vi "FT10_Connect M4X.vi"(8 "error in (no error)":errorcluster, 9 "reset device":bool=TRUE, 10 "Board #":u32, 11 "Message Handling Cluster in":T1={"Fornax Connected?"=refnum, "Unitherm Connected?"=refnum, "M4X Connected?"=refnum, "Unitherm Connect/Disconnect"=refnum, "Fornax Connection"=refnum, "UNITHERM Connection"="", "M4X Connection"=0, "PXI-7854R FPGA Reference"=refnum, "PXI-7854R Connected?"=refnum, "Fornax Connect/Disconnect"=refnum, "7854 Connect/Disconnect"=refnum, "M4X Connect/Disconnect"=refnum, "Config Cluster"={"Unitherm Port"="COM4", "Simulate Values"=TRUE}, "Log Queue"=refnum, "Log Analysis Cluster"={"RMS"=0.0, "Envelope Frequency"=0.0, "Peak"=0.0, "Crest Factor"=0.0, "Duty Cyle %"=0.0, "P-P"=0.0, "Frequency"=0.0, "THD"=0.0, "Postive Peak"=0.0, "Negative Peak"=0.0, "Mag_H1"=0.0, "Phase_H1"=0.0, "Mag_H3"=0.0, "Phase_H3"=0.0, "Mag_H5"=0.0, "Phase_H5"=0.0}, "Log Waveform Cluster"={"t0"=timestamp(0 s since 1904-01-01), "dt"=1.0, "Y"=[]}, "Log Time"=timestamp(0 s since 1904-01-01), "Log Flag"=FALSE}) -> (0 "error out":errorcluster, 1 "M4X Connected?":bool, 2 "Card Handle":u32, 3 "Message Handling Cluster out":T1={"Fornax Connected?"=refnum, "Unitherm Connected?"=refnum, "M4X Connected?"=refnum, "Unitherm Connect/Disconnect"=refnum, "Fornax Connection"=refnum, "UNITHERM Connection"="", "M4X Connection"=0, "PXI-7854R FPGA Reference"=refnum, "PXI-7854R Connected?"=refnum, "Fornax Connect/Disconnect"=refnum, "7854 Connect/Disconnect"=refnum, "M4X Connect/Disconnect"=refnum, "Config Cluster"={"Unitherm Port"="COM4", "Simulate Values"=TRUE}, "Log Queue"=refnum, "Log Analysis Cluster"={"RMS"=0.0, "Envelope Frequency"=0.0, "Peak"=0.0, "Crest Factor"=0.0, "Duty Cyle %"=0.0, "P-P"=0.0, "Frequency"=0.0, "THD"=0.0, "Postive Peak"=0.0, "Negative Peak"=0.0, "Mag_H1"=0.0, "Phase_H1"=0.0, "Mag_H3"=0.0, "Phase_H3"=0.0, "Mag_H5"=0.0, "Phase_H5"=0.0}, "Log Waveform Cluster"={"t0"=timestamp(0 s since 1904-01-01), "dt"=1.0, "Y"=[]}, "Log Time"=timestamp(0 s since 1904-01-01), "Log Flag"=FALSE})   [LabVIEW 2015]
doc: "Copy of \"FT10_Connect M4X.vi\" from HWT_Lillis_7854.lvproj"
uses:
  Controls/Control_Message Handling Cluster.ctl
  Controls/Control_M4X Connection.ctl
  Controls/Control_PXI-7854R FPGA Reference.ctl
  Controls/Control_Config Cluster.ctl
  Controls/Control_Config Unitherm Port.ctl
  Controls/Control_Config Simulate Values.ctl
  Controls/Control_Log Queue.ctl
  Controls/Control_Log Cluster.ctl
  Controls/Control_Log Time.ctl
  Controls/Control_Log Waveform Cluster.ctl
  Controls/Control_Log Analysis Cluster.ctl
  Controls/Control_Log Flag.ctl
  spcm_win32.dll
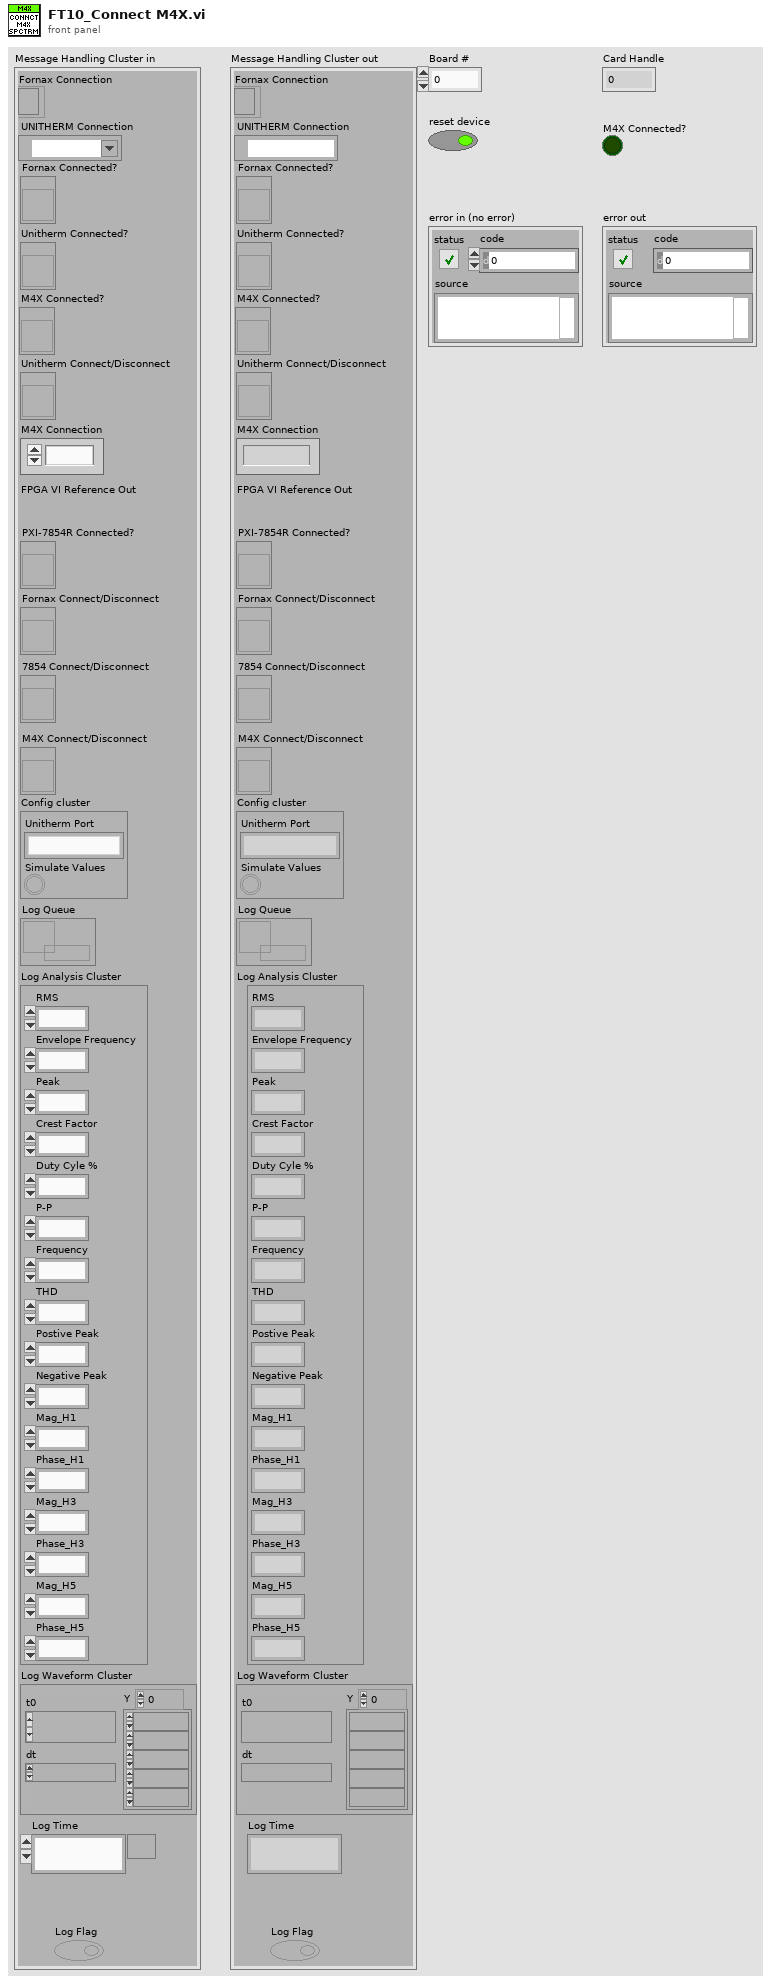
[diagram p1: front panel]
types:
  T1 = typedef "Control_Message Handling Cluster.ctl" = cluster{"Fornax Connected?":refnum<vi>, "Unitherm Connected?":refnum<vi>, "M4X Connected?":refnum<vi>, "Unitherm Connect/Disconnect":refnum<vi>, "Fornax Connection":refnum<k5>, "UNITHERM Connection":refnum<visa-resource-name>, "M4X Connection":T2, "PXI-7854R FPGA Reference":T3, "PXI-7854R Connected?":refnum<vi>, "Fornax Connect/Disconnect":refnum<vi>, "7854 Connect/Disconnect":refnum<vi>, "M4X Connect/Disconnect":refnum<vi>, "Config Cluster":T4, "Log Queue":T7, "Log Analysis Cluster":T8, "Log Waveform Cluster":T9, "Log Time":T10, "Log Flag":T11}
  T2 = typedef "Control_M4X Connection.ctl" = u32
  T3 = typedef "Control_PXI-7854R FPGA Reference.ctl" = refnum<k20>
  T4 = typedef "Control_Config Cluster.ctl" = cluster{"Unitherm Port":T5, "Simulate Values":T6}
  T5 = typedef "Control_Config Unitherm Port.ctl" = string
  T6 = typedef "Control_Config Simulate Values.ctl" = bool
  T7 = typedef "Control_Log Queue.ctl" = refnum<queue>
  T8 = typedef "Control_Log Analysis Cluster.ctl" = cluster{"RMS":dbl, "Envelope Frequency":dbl, "Peak":dbl, "Crest Factor":dbl, "Duty Cyle %":dbl, "P-P":dbl, "Frequency":dbl, "THD":dbl, "Postive Peak":dbl, "Negative Peak":dbl, "Mag_H1":dbl, "Phase_H1":dbl, "Mag_H3":dbl, "Phase_H3":dbl, "Mag_H5":dbl, "Phase_H5":dbl}
  T9 = typedef "Control_Log Waveform Cluster.ctl" = waveform(dbl)
  T10 = typedef "Control_Log Time.ctl" = timestamp
  T11 = typedef "Control_Log Flag.ctl" = bool
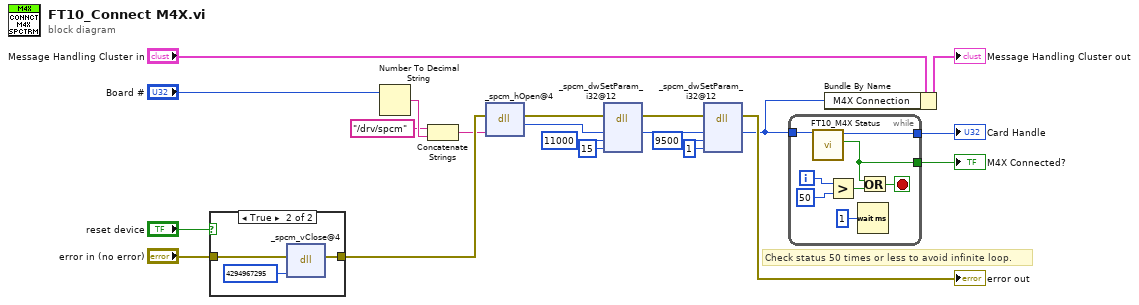
[diagram p0: block diagram]
diagram:
  # "Check status 50 times or less to avoid infinite loop."
  n1 = case shown="True" "reset device" {
    tunnel: "error in (no error)" -> [w22 w25]
    tunnel: [w22 w24] -> w10
    frame False {
    }
    frame True {
      n2 = dll-call lib="spcm_win32.dll" fn="_spcm_vClose@4"(error in=w25, "hDrv"=u32 4294967295) -> (error out=w24:errorcluster)  [unwired: 4 in, 1 out]
    }
  }
  n3 = Number To Decimal String(number="Board #") -> (decimal integer string=w8:string)  [unwired: 1 in]
  n4 = Concatenate Strings("/drv/spcm" ("szDeviceName"), w8) -> (w7:string)
  n5 = dll-call lib="spcm_win32.dll" fn="_spcm_hOpen@4"(error in=w10, "szDeviceName"=w7) -> (error out=w12:errorcluster, "hDrv"=w13:u32)  [unwired: 3 in, 1 out]
  n6 = dll-call lib="spcm_win32.dll" fn="_spcm_dwSetParam_i32@12" label="SPC_CHENABLE"(error in=w12, "hDrv"=w13, "lRegister"=11000, "lValue"=15) -> (error out=w16:errorcluster, "hDrv"=w17:u32)  [unwired: 5 in, 1 out]
  n7 = dll-call lib="spcm_win32.dll" fn="_spcm_dwSetParam_i32@12" label="SPC_CARDMODE"(error in=w16, "hDrv"=w17, "lRegister"=9500, "lValue"=1) -> (error out=→"error out":errorcluster, "hDrv"=w3:u32)  [unwired: 5 in, 1 out]
  n8 = while {
    tunnel: w3 -> [w32]
    tunnel: [w31] -> w2
    tunnel: [w26] -> w1
    i -> [w30]
    stop <- w28 stop-if-true
    n9 = call "FT10_M4X Status.vi"("Card Handle in"=w32) -> ("Ready?"=w26:bool, "Card Handle out"=w31:u32)  [unwired: 9 in]
    n10 = Greater?(x=w30, y=50) -> (0:w27:bool)
    n11 = Wait (ms)(milliseconds to wait=u32 1) -> ()  [unwired: 1 out]
    n12 = Or(x=w26, y=w27) -> (x .or. y?=w28:bool)
  }
  "Card Handle" <- w2
  "M4X Connected?" <- w1
  n13 = Bundle By Name(cluster="Message Handling Cluster in", "M4X Connection"=w3) -> (→"Message Handling Cluster out":T1)
